vi "Photon-STR18.vi"() -> ()   [LabVIEW 2017]
uses:
  programas finales/Menu.ctl
  <vilib>/Analysis/baseanly.llb/Mean (DBL).vi
  <vilib>/Utility/file.llb/Write Delimited Spreadsheet (DBL).vi
  <vilib>/Analysis/NI_AALBase.lvlib
panel:
  in  "EXIT":bool
  in  "Save Data":bool
  in  "Open File":bool
  in  "P":i32=64
  out "Numeric":i32
  out "sum A":dbl format="%#_10g"
  out "sum B":dbl format="%#_10g"
  out "Correlacion":cluster{ext[], ext[]}(graph)
  out "# of Channels":i32
  out "Duration":sgl
  in  "m":i32=2
  out "time":ext[](array[numeric])
  out "corr":ext[](array[numeric])
  out "d*(k)":dbl[][](array[numeric])
  out "Structura":cluster{ext[], ext[]}(graph)
  out "x2 A out":dbl[][](array[numeric])
  out "x2 B out":dbl[][](array[numeric])
  out "g(k) lineal":ext[](array[numeric])
  out "millisecond timer value":u32
  in  "Mode 2":u16(ring)=1 items=["Lineal correlation", "Multi-tau correlation"]
  in  "Data type":u16(ring) items=["Ascii", "Binary"]
  in  "Sample  time (a.u.)":sgl=1000.0
  out "segmentation ChA":sgl[](array[numeric])
  out "tau":dbl[](array[numeric]) format="%#_12g"
  out "sum ChA":sgl format="%#_10g"
  out "Duration A [s]":dbl
  out "tau 3":dbl[](array[numeric]) format="%#_10g"
  out "Segmentation ChB 2":sgl[](array[numeric])
  out "Duration B [s] 2":dbl
  out "tamaño B 2":i32
  out "tau 2":dbl[](array[numeric]) format="%#_10g"
  out "Segmentation ChB":sgl[](array[numeric])
  out "sum ChB":sgl format="%#_10g"
  out "Duration B [s]":dbl
  out "Size B":i32
  out "Size A":i32
  out "Max photon CHA":i32
  out "size(s) 2":i32
  out "time out":dbl[](array[numeric]) format="%#_10g"
  out "Max photon CHB 3":i32
  out "Max photon CHB":i32
  out "CHA":u8[](array[numeric])
  out "CHB":u8[](array[numeric])
  in  "Half data":bool
  out "size(s) 3":i32
  in  "Analysis":u16(ring) items=["Auto correlation A", "Auto correlation B", "Cross correlation AxB", "Cross correlation BxA"]
  out "elapsed time in min":dbl
  out "Elapsed time (s)":dbl
  # "PhotonSTR-18"
  # "Parameters"
  # "Duration A"
  # "Total # of photons A"
  # "Channel A"
  # "Duration B"
  # "Total # of photons B"
  # "Operation Mode"
  # "Channel B"
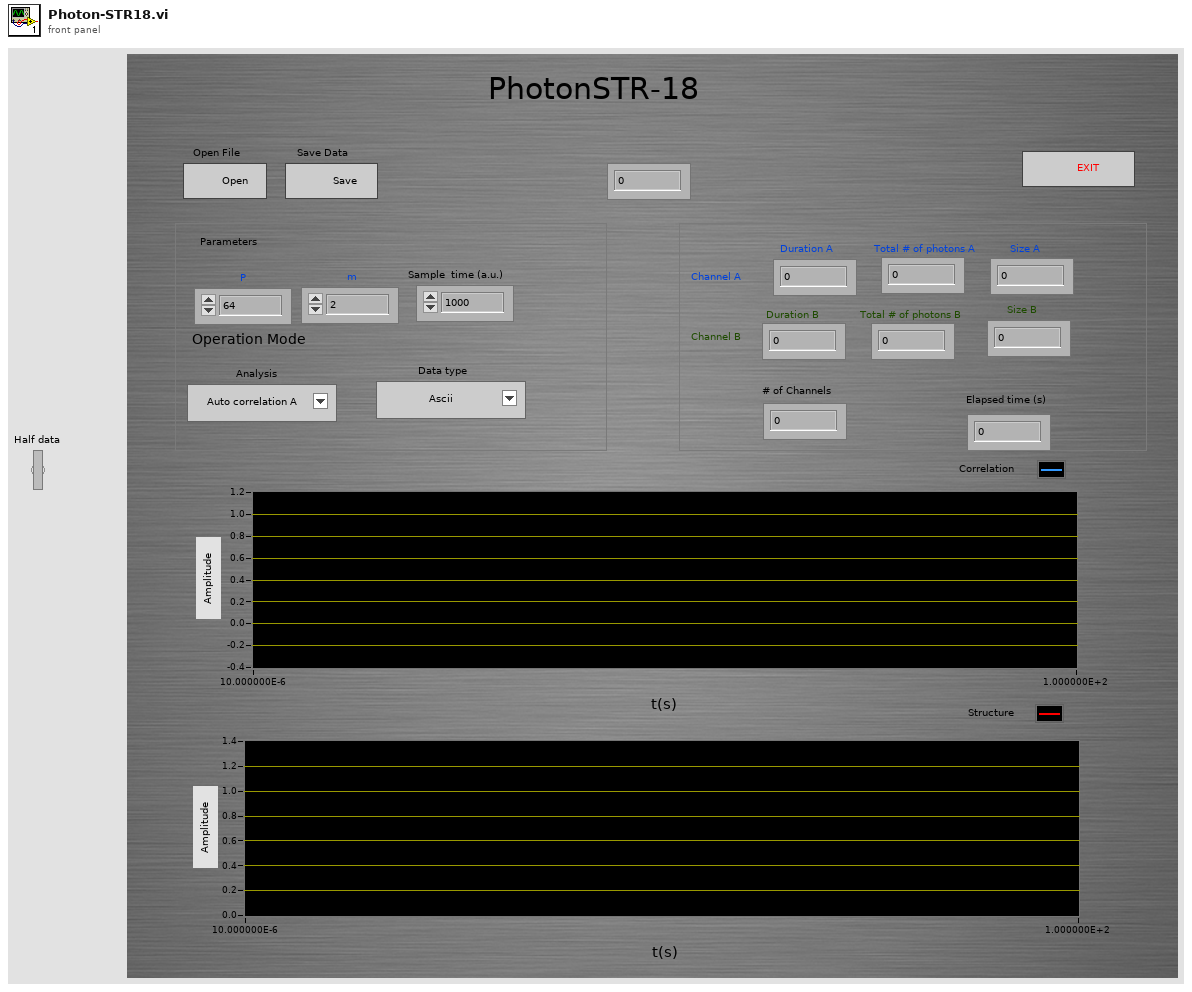
[diagram p1: front panel]
types:
  T1 = typedef "Menu.ctl" = enum16{"Init", "user action", "Load file", "Select range", "Process Photons(t)", "Process Segmentation", "Process Correlation ", "Save data", "Stop"}
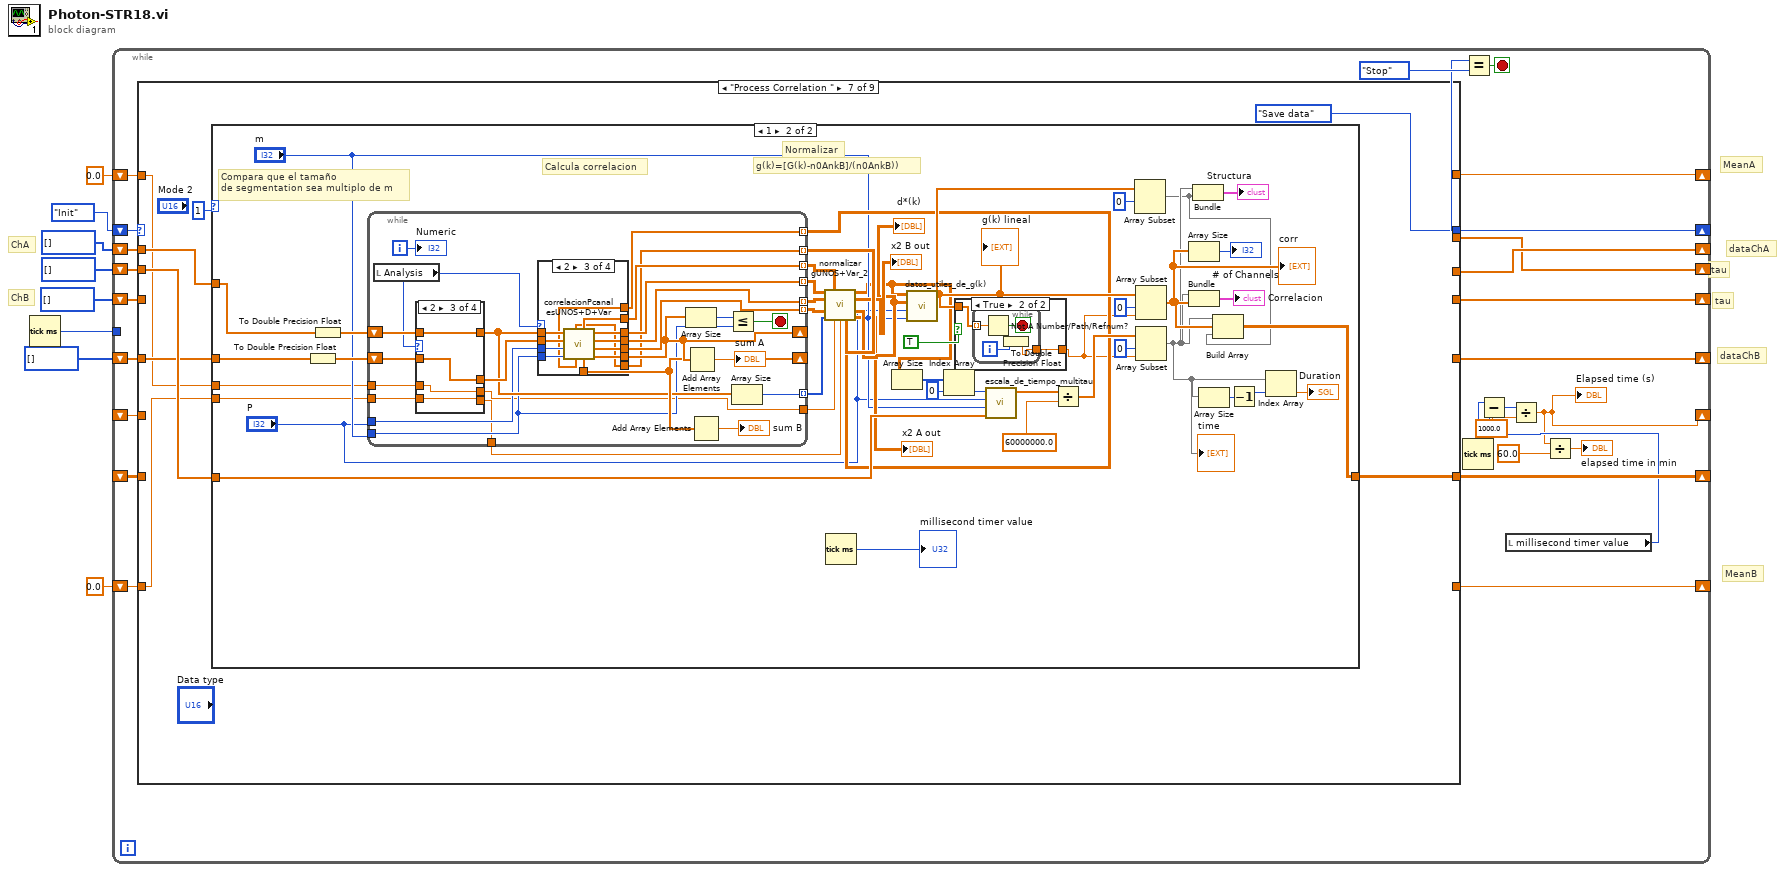
[diagram p0: block diagram]
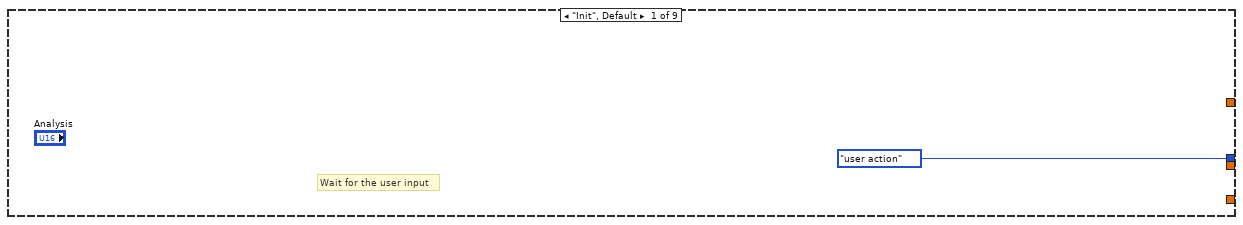
[diagram p2: hidden frame]
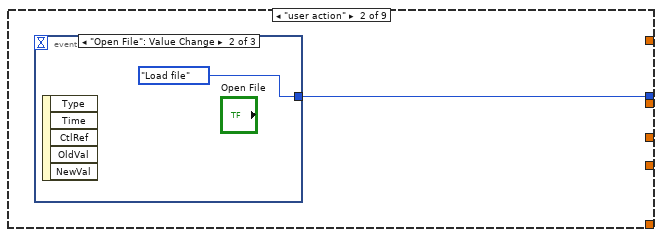
[diagram p3: hidden frame]
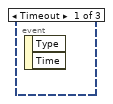
[diagram p4: hidden frame]
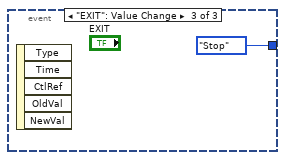
[diagram p5: hidden frame]
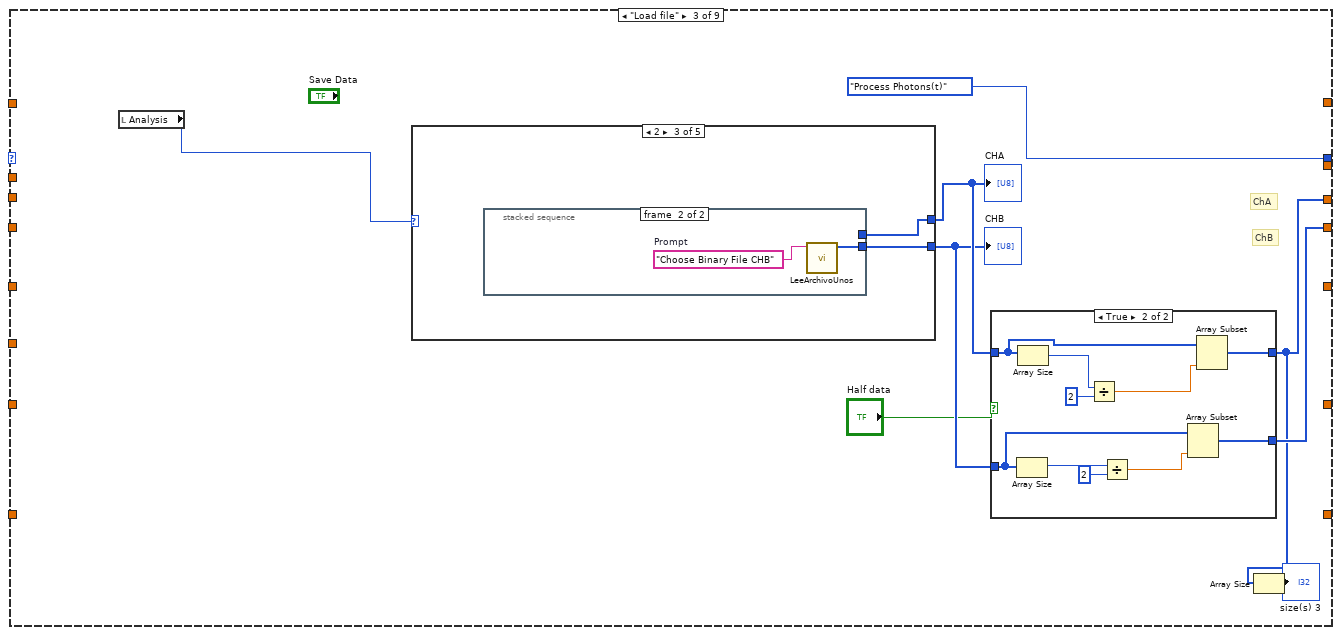
[diagram p6: hidden frame]
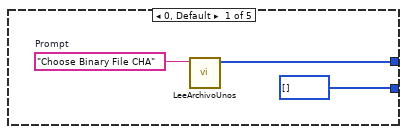
[diagram p8: hidden frame]
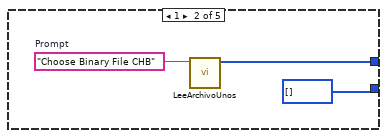
[diagram p9: hidden frame]
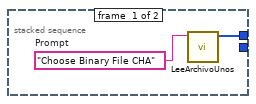
[diagram p10: hidden frame]
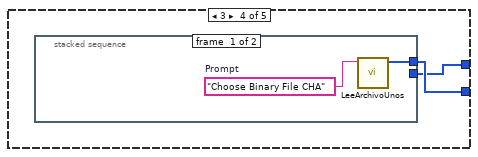
[diagram p11: hidden frame]
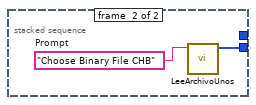
[diagram p12: hidden frame]
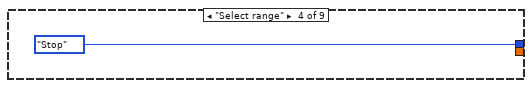
[diagram p14: hidden frame]
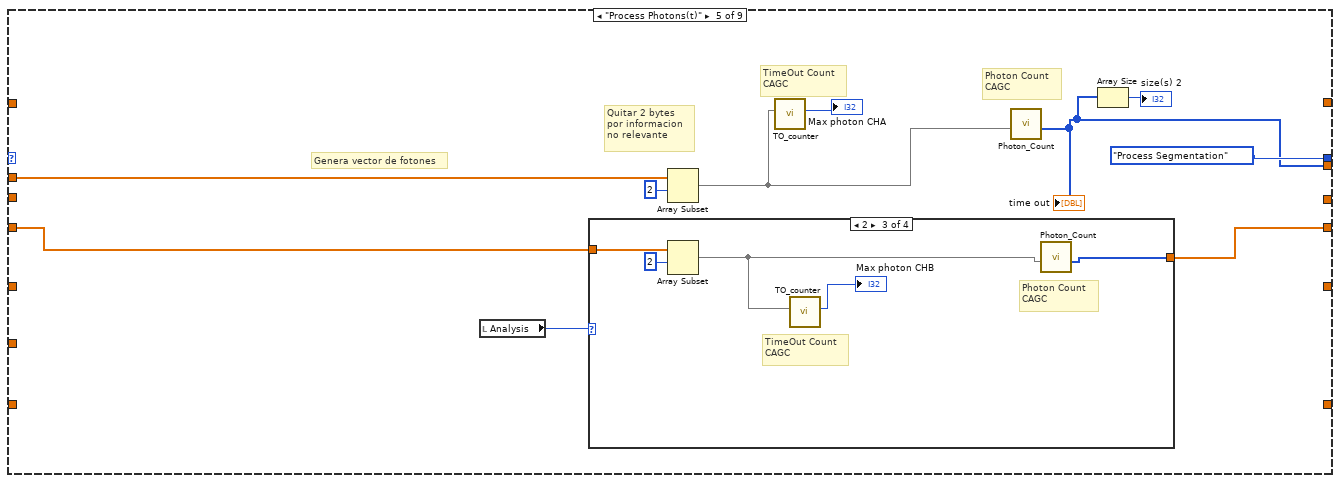
[diagram p15: hidden frame]
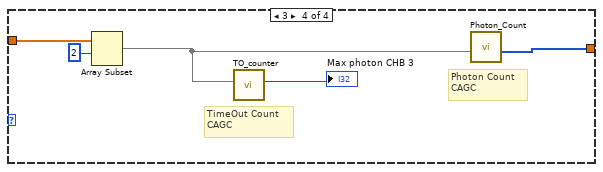
[diagram p18: hidden frame]
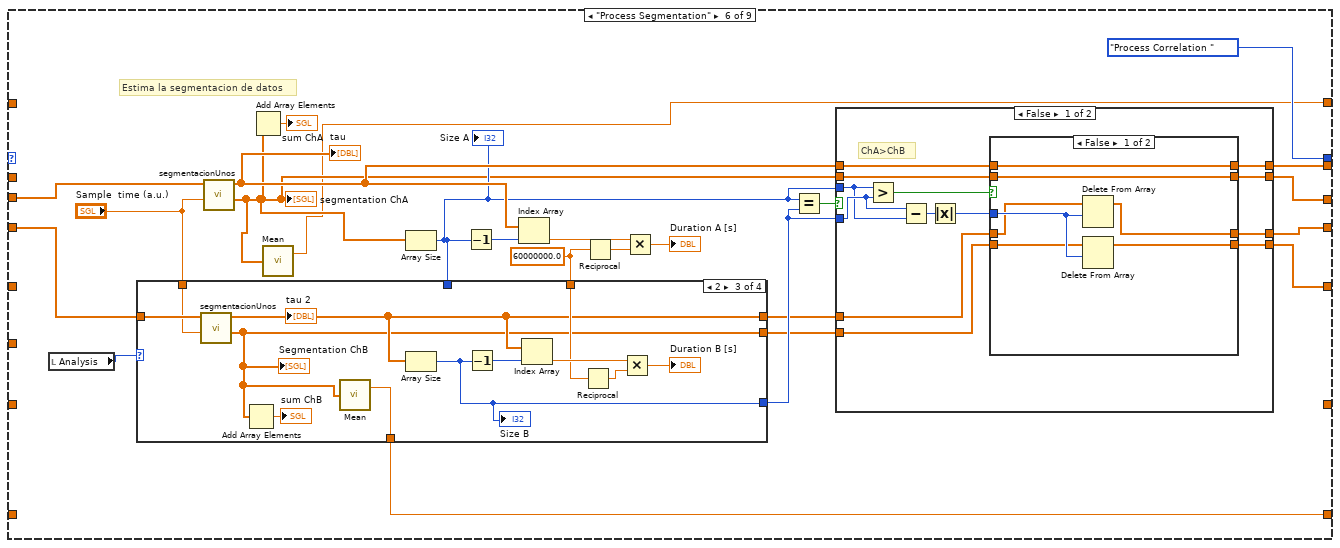
[diagram p19: hidden frame]
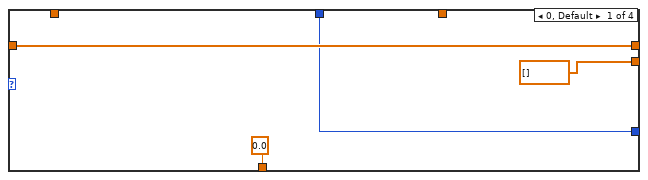
[diagram p20: hidden frame]
diagram:
  # "MeanB"
  # "MeanA"
  # "tau"
  # "tau"
  # "ChB"
  # "dataChB"
  # "dataChA"
  # "ChA"
  n1 = Tick Count (ms)() -> (millisecond timer value=w5:u32)
  n2 = while {
    shift-right: [w32] -> _
    shift-left: Menu."Init" ("Menu") -> [w34]
    shift-right: [w30] -> _
    shift-left: u32[] [] ("Photon trace A") -> [w29]
    shift-right: [w28] -> _
    shift-left: u32[] [] ("Photon trace A") -> [w27]
    shift-right: [w16] -> _
    shift-left: _ -> [w26]
    tunnel: w5 -> [_]
    shift-right: [w20] -> _
    shift-left: u32[] [] ("Photon trace A") -> [w19]
    shift-right: [w18] -> _
    shift-left: u32[] [] ("Photon trace A") -> [w17]
    shift-right: [w13] -> _
    shift-left: _ -> [w15]
    shift-right: [w12] -> _
    shift-left: 0.0 ("mean") -> [w10]
    shift-right: [w11] -> _
    shift-left: 0.0 ("mean") -> [w9]
    stop <- w31 stop-if-true
    n3 = case shown="\"Process Correlation \"" w34 {
      tunnel: [Menu."user action" ("Menu") w36 Menu."Process Photons(t)" ("Menu") Menu."Stop" ("Menu") Menu."Process Segmentation" ("Menu") Menu."Process Correlation " ("Menu") Menu."Save data" ("Menu") Menu."Stop" ("Menu") Menu."Stop" ("Menu")] -> w32
      tunnel: [_ _ w40 _ _ w109 _ _ _] -> w30
      tunnel: w29 -> [_ _ _ _ w85 _ w190 _ _]
      tunnel: [_ _ _ _ w78 w110 _ _ _] -> w28
      tunnel: w27 -> [_ _ _ _ _ w120 w192 _ _]
      tunnel: [_ _ _ _ _ _ w191 _ _] -> w16
      tunnel: w26 -> [_ _ _ _ _ _ _ w327 _]
      tunnel: [_ _ w41 _ w83 w107 _ _ _] -> w20
      tunnel: w19 -> [_ _ _ _ w84 w121 _ _ _]
      tunnel: [_ _ _ _ _ w105 _ _ _] -> w18
      tunnel: w17 -> [_ _ _ _ _ _ w189 _ _]
      tunnel: w15 -> [_ _ _ _ _ _ _ _ _]
      tunnel: [_ _ _ _ _ w100 _ _ _] -> w12
      tunnel: [_ _ _ _ _ w101 _ _ _] -> w11
      tunnel: w10 -> [_ _ _ _ _ _ w187 _ _]
      tunnel: w9 -> [_ _ _ _ _ _ w186 _ _]
      frame "Init", Default {
        # "Wait for the user input"
      }
      frame "user action" {
        n4 = event shown="[1] \"Open File\": Value Change" {
          selector: _ -> [_ _ _]
          dyn-events: _ -> [_ _ _]
          timeout: _ -> [_ _ _]
          tunnel: [_ Menu."Load file" ("Menu") Menu."Stop" ("Menu")] -> w36
          event Timeout {
            n5 = event-data() -> ()  [unwired: 1 in, 2 out]
          }
          event "Open File": Value Change {
            n6 = event-data() -> ()  [unwired: 1 in, 5 out]
          }
          event "EXIT": Value Change {
            n7 = event-data() -> ()  [unwired: 1 in, 5 out]
          }
        }
      }
      frame "Load file" {
        # "ChB"
        # "ChA"
        n8 = local read "Analysis"() -> (w45:u16)
        n9 = case shown="2" w45 {
          tunnel: [w60 w63 w66 w71 _] -> w44
          tunnel: [u8[] [] u8[] [] w65 w72 _] -> w43
          frame 0, Default {
            w61 = "Choose Binary File CHA"  # Prompt
            n10 = call "LeeArchivoUnos.vi"("prompt"=w61) -> ("Datos"=w60:u8[])  [unwired: 8 in, 2 out]
          }
          frame 1 {
            w64 = "Choose Binary File CHB"  # Prompt
            n11 = call "LeeArchivoUnos.vi"("prompt"=w64) -> ("Datos"=w63:u8[])  [unwired: 8 in, 2 out]
          }
          frame 2 {
            n12 = stacked-sequence {
              tunnel: [w67 _] -> w66
              tunnel: [_ w69] -> w65
              frame #0 {
                w68 = "Choose Binary File CHA"  # Prompt
                n13 = call "LeeArchivoUnos.vi"("prompt"=w68) -> ("Datos"=w67:u8[])  [unwired: 8 in, 2 out]
              }
              frame #1 {
                w70 = "Choose Binary File CHB"  # Prompt
                n14 = call "LeeArchivoUnos.vi"("prompt"=w70) -> ("Datos"=w69:u8[])  [unwired: 8 in, 2 out]
              }
            }
          }
          frame 3 {
            n15 = stacked-sequence {
              tunnel: [w73 _] -> w72
              tunnel: [_ w75] -> w71
              frame #0 {
                w74 = "Choose Binary File CHA"  # Prompt
                n16 = call "LeeArchivoUnos.vi"("prompt"=w74) -> ("Datos"=w73:u8[])  [unwired: 8 in, 2 out]
              }
              frame #1 {
                w76 = "Choose Binary File CHB"  # Prompt
                n17 = call "LeeArchivoUnos.vi"("prompt"=w76) -> ("Datos"=w75:u8[])  [unwired: 8 in, 2 out]
              }
            }
          }
          frame 4 {
          }
        }
        "CHA" <- w44
        "CHB" <- w43
        n18 = case shown="True" "Half data" {
          tunnel: w44 -> [w48 w58]
          tunnel: w43 -> [w47 w57]
          tunnel: [w48 w50] -> w40
          tunnel: [w47 w49] -> w41
          frame False {
          }
          frame True {
            n19 = Array Size(array=w57) -> (size(s)=w55:i32)
            n20 = Array Size(array=w58) -> (size(s)=w56:i32)
            n21 = Divide(x=w56, y=2) -> (x/y=w51:dbl)
            n22 = Divide(x=w55, y=2) -> (x/y=w52:dbl)
            n23 = Array Subset(array=w57, length=w52) -> (w49:u8[])  [unwired: 1 in]
            n24 = Array Subset(array=w58, length=w51) -> (w50:u8[])  [unwired: 1 in]
          }
        }
        n25 = Array Size(array=w40) -> (size(s)=→"size(s) 3":i32)
      }
      frame "Select range" {
      }
      frame "Process Photons(t)" {
        # "Photon Count\nCAGC"
        # "TimeOut Count\nCAGC"
        # "Quitar 2 bytes\npor informacion\nno relevante"
        # "Genera vector de fotones"
        n26 = local read "Analysis"() -> (w81:u16)
        n27 = case shown="2" w81 {
          tunnel: w84 -> [w88 w89 w93 w98]
          tunnel: [w88 w89 w90 w96] -> w83
          frame 0, Default {
          }
          frame 1 {
          }
          frame 2 {
            # "Photon Count\nCAGC"
            # "TimeOut Count\nCAGC"
            n28 = Array Subset(array=w93, index=2) -> (w91:dbl[])  [unwired: 1 in]
            n29 = call "TO_counter.vi"("Datos"=w91) -> ("Numeric"=→"Max photon CHB":i32)  [unwired: 10 in]
            n30 = call "Photon_Count.vi"("Data in"=w91) -> ("Time out"=w90:i32[])  [unwired: 10 in]
          }
          frame 3 {
            # "Photon Count\nCAGC"
            # "TimeOut Count \nCAGC"
            n31 = Array Subset(array=w98, index=2) -> (w95:dbl[])  [unwired: 1 in]
            n32 = call "TO_counter.vi"("Datos"=w95) -> ("Numeric"=→"Max photon CHB 3":i32)  [unwired: 10 in]
            n33 = call "Photon_Count.vi"("Data in"=w95) -> ("Time out"=w96:i32[])  [unwired: 10 in]
          }
        }
        n34 = Array Subset(array=w85, index=2) -> (w79:sgl[])  [unwired: 1 in]
        n35 = call "TO_counter.vi"("Datos"=w79) -> ("Numeric"=→"Max photon CHA":i32)  [unwired: 10 in]
        n36 = call "Photon_Count.vi"("Data in"=w79) -> ("Time out"=w78:i32[])  [unwired: 10 in]
        "time out" <- w78
        n37 = Array Size(array=w78) -> (size(s)=→"size(s) 2":i32)
      }
      frame "Process Segmentation" {
        w114 = 60000000.0 ("x")
        # "Estima la segmentacion de datos"
        n38 = local read "Analysis"() -> (w104:u16)
        n39 = call "segmentacionUnos.vi"("sample time"="Sample  time (a.u.)", "relative time"=w120) -> ("Segmentation"=w102:sgl[], "tau"=w111:dbl[])  [unwired: 8 in]
        "segmentation ChA" <- w102
        "tau" <- w111
        n40 = Add Array Elements(numeric array=w102) -> (sum=→"sum ChA":sgl)
        n41 = call-poly <vilib>:"Mean.vi"("X"=w102) -> ("mean"=w100:dbl)  [unwired: 1 out]
        n42 = Array Size(array=w102) -> (size(s)=w103:i32)
        "Size A" <- w103
        n43 = case shown="2" w104 {
          tunnel: w121 -> [w127 w130 w142 w150]
          tunnel: "Sample  time (a.u.)" -> [_ _ w141 w149]
          tunnel: w114 -> [_ _ w136 w148]
          tunnel: [w125 w129 w134 w146] -> w112
          tunnel: [w127 w130 w135 w147] -> w108
          tunnel: [sgl[] [] sgl[] [] w133 w145] -> w106
          tunnel: w103 -> [w125 w129 _ _]
          tunnel: [0.0 ("mean") 0.0 ("mean") w132 w144] -> w101
          frame 0, Default {
          }
          frame 1 {
          }
          frame 2 {
            n44 = call "segmentacionUnos.vi"("sample time"=w141, "relative time"=w142) -> ("Segmentation"=w133:sgl[], "tau"=w135:dbl[])  [unwired: 8 in]
            "tau 2" <- w135
            "Segmentation ChB" <- w133
            n45 = Add Array Elements(numeric array=w133) -> (sum=→"sum ChB":sgl)
            n46 = call-poly <vilib>:"Mean.vi"("X"=w133) -> ("mean"=w132:dbl)  [unwired: 1 out]
            n47 = Array Size(array=w135) -> (size(s)=w134:i32)
            "Size B" <- w134
            n48 = Decrement(x=w134) -> (x-1=w140:i32)
            n49 = Index Array(array=w135, index=w140) -> (element=w139:dbl)
            n50 = Reciprocal(x=w136) -> (1/x=w138:dbl)
            n51 = Multiply(x=w139, y=w138) -> (x*y=→"Duration B [s]":dbl)
          }
          frame 3 {
            n52 = call "segmentacionUnos.vi"("sample time"=w149, "relative time"=w150) -> ("Segmentation"=w145:sgl[], "tau"=w147:dbl[])  [unwired: 8 in]
            "tau 3" <- w147
            "Segmentation ChB 2" <- w145
            n53 = call-poly <vilib>:"Mean.vi"("X"=w145) -> ("mean"=w144:dbl)  [unwired: 1 out]
            n54 = Array Size(array=w147) -> (size(s)=w146:i32)
            "tamaño B 2" <- w146
            n55 = Decrement(x=w146) -> (x-1=w154:i32)
            n56 = Index Array(array=w147, index=w154) -> (element=w153:dbl)
            n57 = Reciprocal(x=w148) -> (1/x=w152:dbl)
            n58 = Multiply(x=w153, y=w152) -> (x*y=→"Duration B [s] 2":dbl)
          }
        }
        n59 = Decrement(x=w103) -> (x-1=w118:i32)
        n60 = Index Array(array=w111, index=w118) -> (element=w115:dbl)
        n61 = Reciprocal(x=w114) -> (1/x=w117:dbl)
        n62 = Multiply(x=w115, y=w117) -> (x*y=→"Duration A [s]":dbl)
        n63 = Equal?(x=w103, y=w112) -> (x = y?=w113:bool)
        n64 = case shown="False" w113 {
          tunnel: w111 -> [w163 w185]
          tunnel: w102 -> [w162 w184]
          tunnel: w108 -> [w159 w183]
          tunnel: w106 -> [w160 w182]
          tunnel: w103 -> [w166 _]
          tunnel: w112 -> [w167 _]
          tunnel: [w158 w185] -> w110
          tunnel: [w157 w184] -> w109
          tunnel: [w156 w183] -> w107
          tunnel: [w155 w182] -> w105
          frame False {
            # "ChA>ChB"
            n65 = Greater?(x=w166, y=w167) -> (0:w164:bool)
            n66 = Subtract(x=w167, y=w166) -> (x-y=w165:i32)
            n67 = Absolute Value(x=w165) -> (abs(x)=w161:i32)
            n68 = case shown="False" w164 {
              tunnel: w163 -> [w169 w181]
              tunnel: w162 -> [w168 w180]
              tunnel: w161 -> [w174 w179]
              tunnel: [w169 w178] -> w158
              tunnel: [w168 w177] -> w157
              tunnel: w160 -> [w172 w175]
              tunnel: w159 -> [w173 w176]
              tunnel: [w170 w176] -> w156
              tunnel: [w171 w175] -> w155
              frame False {
                n69 = Delete From Array(array=w173, length=w174) -> (array with subset deleted=w170:dbl[])  [unwired: 1 in, 1 out]
                n70 = Delete From Array(array=w172, length=w174) -> (array with subset deleted=w171:sgl[])  [unwired: 1 in, 1 out]
              }
              frame True {
                n71 = Delete From Array(array=w181, length=w179) -> (array with subset deleted=w178:dbl[])  [unwired: 1 in, 1 out]
                n72 = Delete From Array(array=w180, length=w179) -> (array with subset deleted=w177:sgl[])  [unwired: 1 in, 1 out]
              }
            }
          }
          frame True {
          }
        }
      }
      frame "Process Correlation " {
        n73 = case shown="1" u16 1 ("Mode 2") {
          tunnel: w192 -> [_ w226]
          tunnel: [_ w228] -> w191
          tunnel: w190 -> [_ w224]
          tunnel: w189 -> [_ w222]
          tunnel: w187 -> [_ w197]
          tunnel: w186 -> [_ w196]
          frame 0, Default {
          }
          frame 1 {
            # "Calcula correlacion"
            # "g(k)=[G(k)-n0AnkB]/(n0AnkB))"
            # "Normalizar"
            # "Compara que el tamaño\nde segmentation sea multiplo de m"
            n74 = To Double Precision Float(number=w222) -> (double precision float=w221:dbl[])
            n75 = To Double Precision Float(number=w224) -> (double precision float=w223:dbl[])
            n76 = while {
              tunnel: [w269] -> w212 mode=indexing
              shift-right: [w265] -> _
              shift-left: w223 -> [w261]
              tunnel: "m" -> [w254]
              tunnel: "P" -> [w256]
              tunnel: [w270] -> w205 mode=indexing
              tunnel: [w271] -> w211 mode=indexing
              tunnel: [w267] -> w210 mode=indexing
              shift-right: [w262] -> _
              shift-left: w221 -> [w260]
              tunnel: [w255] -> w213 mode=indexing
              tunnel: [w253] -> w214 mode=indexing
              tunnel: [w252] -> w206 mode=indexing
              tunnel: w197 -> [w251]
              tunnel: w196 -> [w250]
              tunnel: [w249] -> w195
              tunnel: [w248] -> w194
              i -> [w266]
              stop <- w272 stop-if-true
              n77 = local read "Analysis"() -> (w257:u16)
              n78 = case shown="2" w257 {
                tunnel: w261 -> [w316 w318 w322 w326]
                tunnel: [w316 w318 w322 w326] -> w258
                tunnel: [w316 w318 w321 w325] -> w259
                tunnel: w260 -> [_ _ w321 w325]
                tunnel: w251 -> [w315 w317 w320 w324]
                tunnel: w250 -> [_ _ w319 w323]
                tunnel: [w315 w317 w320 w324] -> w249
                tunnel: [w315 w317 w319 w323] -> w248
                frame 0, Default {
                }
                frame 1 {
                }
                frame 2 {
                }
                frame 3 {
                }
              }
              n79 = case shown="2" w257 {
                tunnel: [w280 w289 w302 w313] -> w271
                tunnel: [w279 w288 w301 w312] -> w270
                tunnel: [w281 w290 w300 w314] -> w269
                tunnel: w256 -> [w277 w286 w299 w307]
                tunnel: w254 -> [w276 w285 w298 w306]
                tunnel: [w275 w284 w297 w311] -> w265
                tunnel: [w275 w284 w296 w310] -> w262
                tunnel: w259 -> [_ _ w295 w308]
                tunnel: w258 -> [w278 w287 w294 w309]
                tunnel: [w274 w283 w293 w305] -> w255
                tunnel: [w273 w282 w292 w304] -> w253
                tunnel: [w273 w282 w291 w303] -> w252
                frame 0, Default {
                  n80 = call "correlacionPcanales+D+Var.vi"("m"=w276, "P"=w277, "input A"=w278) -> ("Sn"=w275:dbl[], "MonitorX out"=w279:dbl[], "MonitorY out"=w280:dbl[], "Acc"=w281:dbl[], "x2 out"=w273:dbl[], "Acc D"=w274:dbl[])  [unwired: 3 in]
                }
                frame 1 {
                  n81 = call "correlacionPcanales+D+Var.vi"("m"=w285, "P"=w286, "input A"=w287) -> ("Sn"=w284:dbl[], "MonitorX out"=w288:dbl[], "MonitorY out"=w289:dbl[], "Acc"=w290:dbl[], "x2 out"=w282:dbl[], "Acc D"=w283:dbl[])  [unwired: 3 in]
                }
                frame 2 {
                  n82 = call "correlacionPcanalesUNOS+D+Var.vi"("m"=w298, "P"=w299, "input B"=w295, "input A"=w294) -> ("Sn A"=w297:dbl[], "MonitorX out"=w301:dbl[], "MonitorY out"=w302:dbl[], "Acc"=w300:dbl[], "Sn B"=w296:dbl[], "Acc D"=w293:dbl[], "x2 B out"=w291:dbl[], "x2 A out"=w292:dbl[])
                }
                frame 3 {
                  n83 = call "correlacionPcanalesUNOS+D+Var.vi"("m"=w306, "P"=w307, "input B"=w308, "input A"=w309) -> ("Sn A"=w311:dbl[], "MonitorX out"=w312:dbl[], "MonitorY out"=w313:dbl[], "Acc"=w314:dbl[], "Sn B"=w310:dbl[], "Acc D"=w305:dbl[], "x2 B out"=w303:dbl[], "x2 A out"=w304:dbl[])
                }
              }
              n84 = Array Size(array=w265) -> (size(s)=w268:i32)
              n85 = Add Array Elements(numeric array=w265) -> (sum=→"sum A":dbl)
              n86 = Add Array Elements(numeric array=w262) -> (sum=→"sum B":dbl)
              n87 = Less Or Equal?(x=w268, y=w254) -> (x <= y?=w272:bool)
              n88 = Array Size(array=w258) -> (size(s)=w267:i32)
              "Numeric" <- w266
            }
            n89 = call "normalizar gUNOS+Var_2.vi"("Acc"=w212, "Acc D"=w213, "x2 A in"=w214, "MonitorY out"=w211, "MonitorX out"=w205, "Tamaño Sn"=w210, "AvgA"=w195, "AvgB"=w194, "x2 B in"=w206) -> ("g(k)"=w202:dbl[][], "x2 B out"=→"x2 B out":dbl[][], "d*(k)"=w208:dbl[][], "x2 A out"=→"x2 A out":dbl[][])  [unwired: 1 in, 2 out]
            "d*(k)" <- w208
            n90 = Tick Count (ms)() -> (millisecond timer value=→"millisecond timer value":u32)
            n91 = Array Size(array=w202) -> (size(s)=w239:i32[])
            n92 = call "datos_utiles_de_g(k) .vi"("m"="m", "P"="P", "d(k) in"=w208, "g(k) in"=w202) -> ("d(k) lineal"=w216:ext[], "g(k) lineal"=w219:ext[])  [unwired: 6 in]
            "g(k) lineal" <- w219
            n93 = Index Array(array=w239, index=0) -> (element=w227:i32)
            n94 = case shown="True" TRUE {
              tunnel: w219 -> [w241 w243]
              tunnel: [w240 w242] -> w200
              frame False {
                n95 = Array Size(array=w241) -> (size(s)=w240:i32)
              }
              frame True {
                n96 = while {
                  tunnel: w243 -> [w247] mode=indexing
                  tunnel: [w244] -> w242
                  i -> [w245]
                  stop <- w246 stop-if-true
                  n97 = Not A Number/Path/Refnum?(number/path/refnum=w247) -> (NaN/Path/Refnum?=w246:bool)
                  n98 = To Double Precision Float(number=w245) -> (double precision float=w244:dbl)
                }
              }
            }
            n99 = call "escala_de_tiempo_multitau.vi"("tau"=w226, "m"="m", "P"="P", "No. of shift registers"=w227) -> ("time multi-tau"=w225:ext[])  [unwired: 7 in]
            n100 = Divide(x=w225, y=60000000.0) -> (x/y=w230:ext[])
            n101 = Array Subset(array=w216, index=0) -> (w199:ext[])  [unwired: 1 in]
            n102 = Array Subset(array=w219, index=0, length=w200) -> (w220:ext[])
            "corr" <- w220
            n103 = Array Subset(array=w230, index=0, length=w200) -> (w203:ext[])
            "time" <- w203
            n104 = Array Size(array=w220) -> (size(s)=→"# of Channels":i32)
            n105 = Bundle(w203, w220) -> (→"Correlacion":cluster{ext[], ext[]})  [unwired: 1 in]
            n106 = Bundle(w203, w199) -> (→"Structura":cluster{ext[], ext[]})  [unwired: 1 in]
            n107 = Array Size(array=w203) -> (size(s)=w235:i32)
            n108 = Build Array(w203, w220, w199) -> (w228:ext[][])
            n109 = Decrement(x=w235) -> (x-1=w234:i32)
            n110 = Index Array(array=w203, index=w234) -> (element=→"Duration":ext)
          }
        }
      }
      frame "Save data" {
        # "Save data"
        n111 = Two Button Dialog(message="Do you want to save the data?", 1:"No" ("F button name (\"Cancel\")"), 2:"Yes" ("T button name (\"OK\")")) -> (T button?=w328:bool)
        n112 = case shown="True" w328 {
          tunnel: w327 -> [_ w335]
          frame False {
          }
          frame True {
            n113 = Transpose 2D Array(2D array=w335) -> (transposed array=w333:ext[][])
            n114 = call-poly <vilib>:"Write Delimited Spreadsheet.vi"("format (%.3f)"="%.6e", "2D data"=w333) -> ()  [unwired: 12 in, 2 out]
          }
        }
      }
      frame "Stop" {
        # "Registry cleanse"
      }
    }
    n115 = Tick Count (ms)() -> (millisecond timer value=w23:u32)
    n116 = Equal?(x=w32, y=Menu."Stop" ("Menu")) -> (x = y?=w31:bool)
    n117 = local read "millisecond timer value"() -> (w14:u32)
    n118 = Subtract(x=w23, y=w14) -> (x-y=w25:u32)
    n119 = Divide(x=w25, y=1000.0) -> (x/y=w13:dbl)
    "Elapsed time (s)" <- w13
    n120 = Divide(x=w13, y=60.0) -> (x/y=→"elapsed time in min":dbl)
  }
